vi "start.vi"(8 "error in (no error)":errorcluster, 11 "ScanHeadAK130114ResonanceFlexRIO in":refnum<class "ScanHeadAK130114ResonanceFlexRIO.lvclass">) -> (0 "error out":errorcluster, 3 "ScanHeadAK130114ResonanceFlexRIO out":refnum<class "ScanHeadAK130114ResonanceFlexRIO.lvclass">)   [LabVIEW 2010, in "ScanHeadAK130114ResonanceFlexRIO.lvclass"]
uses:
  ScanHeadAK130114ResonanceFlexRIO.lvclass
  Trajectory/GenericTrajectory/GenericTrajectory/GenericTrajectory.lvclass
  Trajectory/TrajectoryMG100122GenericFPGA/TrajectoryMG100122GenericFPGA/TrajectoryMG100122GenericFPGA.lvclass
  common/classes/ErrorController/ErrorController/class_data.vi
  DAQ/GenericDAQ/GenericDAQ/GenericDAQ.lvclass
  common/classes/ErrorController/ErrorController/ErrorController.lvclass
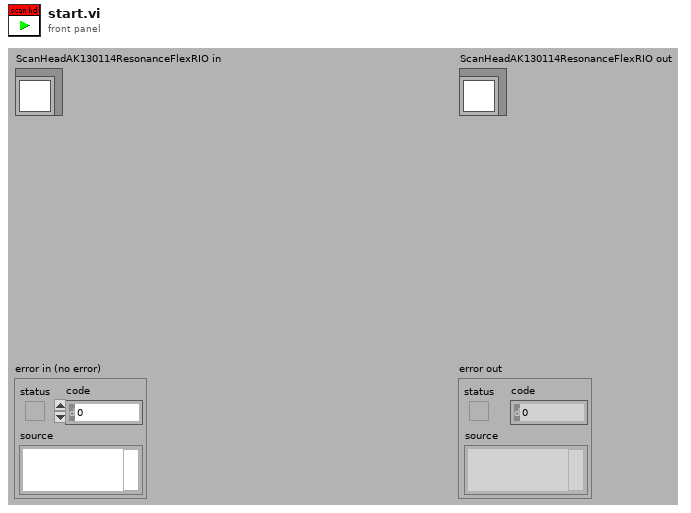
[diagram p1: front panel]
types:
  T1 = typedef "GenericToplevelComponent.lvclass/common_trigger_enum.ctl" = enum16{"NULL", "initialise", "terminate", "fetch command", "fetch data", "attach observer", "register as observer", "detach observer", "acknowledge", "start", "stop", "sweep started", "sweep finished", "experiment started", "experiment stopped"}
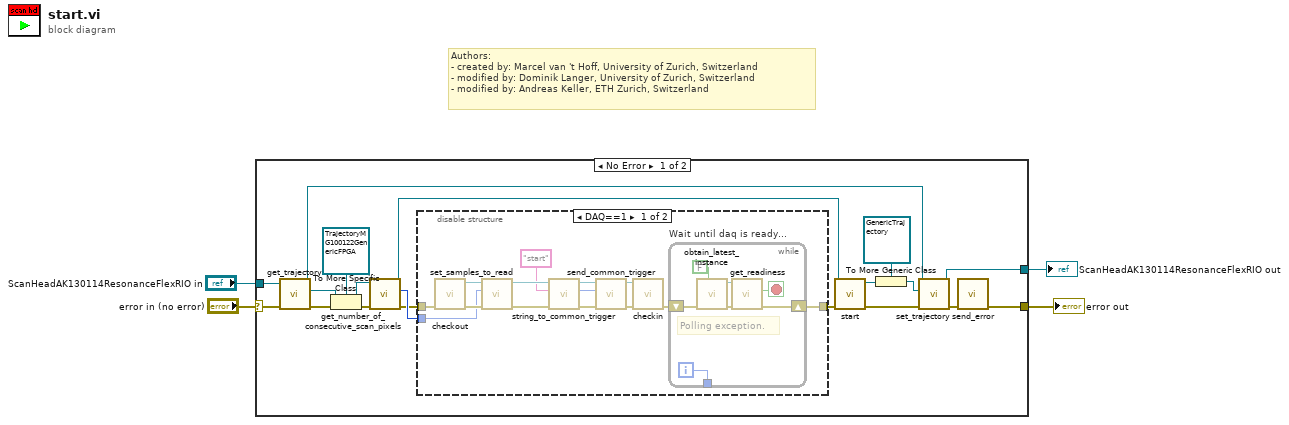
[diagram p0: block diagram]
diagram:
  # "Authors: \n- created by: Marcel van 't Hoff, University of Zurich, Switzerland\n- modified by: Dominik Langer, University of Zurich, Switzerland\n- modified by: Andreas Keller, ETH Zurich, Switzerland"
  n1 = case shown="No Error" "error in (no error)" {
    selector: "error in (no error)" -> [w8 w46]
    tunnel: "ScanHeadAK130114ResonanceFlexRIO in" -> [w7 w47]
    tunnel: [w6 w46] -> w2
    tunnel: [w5 w47] -> w1
    frame No Error {
      n2 = call-dynamic "get_trajectory.vi"("error in (no error)"=w8, "GenericScanHead.lvclass in"=w7) -> ("error out"=w23:errorcluster, "trajectory"=w19:refnum<class "GenericTrajectory.lvclass">, "GenericScanHead.lvclass out"=w20:refnum<class "ScanHeadAK130114ResonanceFlexRIO.lvclass">)  [unwired: 7 in]
      n3 = To More Specific Class(target class=refnum<class "TrajectoryMG100122GenericFPGA.lvclass"> refnum ("TrajectoryMG100122GenericFPGA in"), reference=w19, error in=w23) -> (specific class reference=w16:refnum<class "TrajectoryMG100122GenericFPGA.lvclass">, error out=w17:errorcluster)
      n4 = call-dynamic "get_number_of_consecutive_scan_pixels.vi"("error in (no error)"=w17, "GenericTrajectory in"=w16) -> ("error out"=w12:errorcluster, "number of consecutive scan pixels"=w18:i64, "GenericTrajectory out"=w11:refnum<class "TrajectoryMG100122GenericFPGA.lvclass">)  [unwired: 7 in]
      n5 = disable-structure shown="DAQ==1" {
        disable-tunnel: w12 -> [w37 w45]
        disable-tunnel: [w30 w45] -> w13
        disable-tunnel: w18 -> [w32 _]
        frame condition #0 {
          n6 = call "checkout.vi"("error in (no error)"=w37) -> ("error out"=w35:errorcluster, "GenericDAQ out"=w34:refnum<class "GenericDAQ.lvclass">)  [unwired: 9 in]
          n7 = call-dynamic "set_samples_to_read.vi"("error in (no error)"=w35, "samples to read"=w32, "GenericDAQ.lvclass in"=w34) -> ("error out"=w25:errorcluster, "GenericDAQ.lvclass out"=w28:refnum<class "GenericDAQ.lvclass">)  [unwired: 7 in]
          n8 = call-dynamic "string_to_common_trigger.vi"("error in (no error)"=w25, "trigger string"="start", "GenericToplevelComponent in"=w28) -> ("error out"=w26:errorcluster, "trigger"=w29:T1, "GenericToplevelComponent out"=w27:refnum<class "GenericDAQ.lvclass">)  [unwired: 6 in]
          n9 = call-dynamic "send_common_trigger.vi"("error in (no error)"=w26, "trigger"=w29, "GenericToplevelComponent in"=w27) -> ("error out"=w36:errorcluster, "GenericToplevelComponent out"=w33:refnum<class "GenericDAQ.lvclass">)  [unwired: 6 in, 1 out]
          n10 = call-dynamic "checkin.vi"("error in (no error)"=w36, "GenericDAQ in"=w33) -> ("error out"=w31:errorcluster)  [unwired: 8 in, 1 out]
          n11 = while "Wait until daq is ready..." {
            shift-right: [w40] -> w30
            shift-left: w31 -> [w41]
            tunnel: [w38] -> _
            i -> [w38]
            stop <- w39 stop-if-true
            # "Polling exception."
            n12 = call "obtain_latest_instance.vi"("quick, but maybe outdated?"=FALSE, "error in (no error)"=w41) -> ("error out"=w44:errorcluster, "GenericDAQ out"=w43:refnum<class "GenericDAQ.lvclass">)  [unwired: 8 in]
            n13 = call-dynamic "get_readiness.vi"("error in (no error)"=w44, "GenericDAQ in"=w43) -> ("error out"=w40:errorcluster, "ready?"=w39:bool)  [unwired: 7 in, 1 out]
          }
        }
        frame condition #1 (active) {
        }
      }
      n14 = call-dynamic "start.vi"("error in (no error)"=w13, "TrajectoryMG100122GenericFPGA in"=w11) -> ("error out"=w14:errorcluster, "TrajectoryMG100122GenericFPGA out"=w10:refnum<class "TrajectoryMG100122GenericFPGA.lvclass">)  [unwired: 8 in]
      n15 = To More Generic Class(target class=refnum<class "GenericTrajectory.lvclass"> refnum ("GenericTrajectory.lvclass"), reference=w10) -> (generic class reference=w9:refnum<class "GenericTrajectory.lvclass">)
      n16 = call-dynamic "set_trajectory.vi"("error in (no error)"=w14, "trajectory"=w9, "GenericScanHead.lvclass in"=w20) -> ("error out"=w15:errorcluster, "GenericScanHead.lvclass out"=w5:refnum<class "ScanHeadAK130114ResonanceFlexRIO.lvclass">)  [unwired: 7 in]
      n17 = call "send_error.vi"("error in (no error)"=w15) -> ("error out"=w6:errorcluster)  [unwired: 10 in]
    }
    frame Error {
    }
  }
  "error out" <- w2
  "ScanHeadAK130114ResonanceFlexRIO out" <- w1
